vi "WrapVI.vi"() -> ()   [LabVIEW 2021]
uses:
  <vilib>/Utility/miscctls.llb/LVPositionTypeDef.ctl
panel:
  out "Facade Library Path":path=path "C:/Repositories/LVOS/jsontext Facade/lv-src/jsontext.facade.lvlib"
  in  "source VI":path
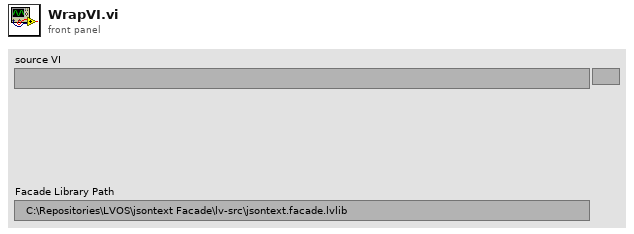
[diagram p1: front panel]
types:
  T1 = typedef "LVPositionTypeDef.ctl" = cluster{"Left":i32, "Top":i32}
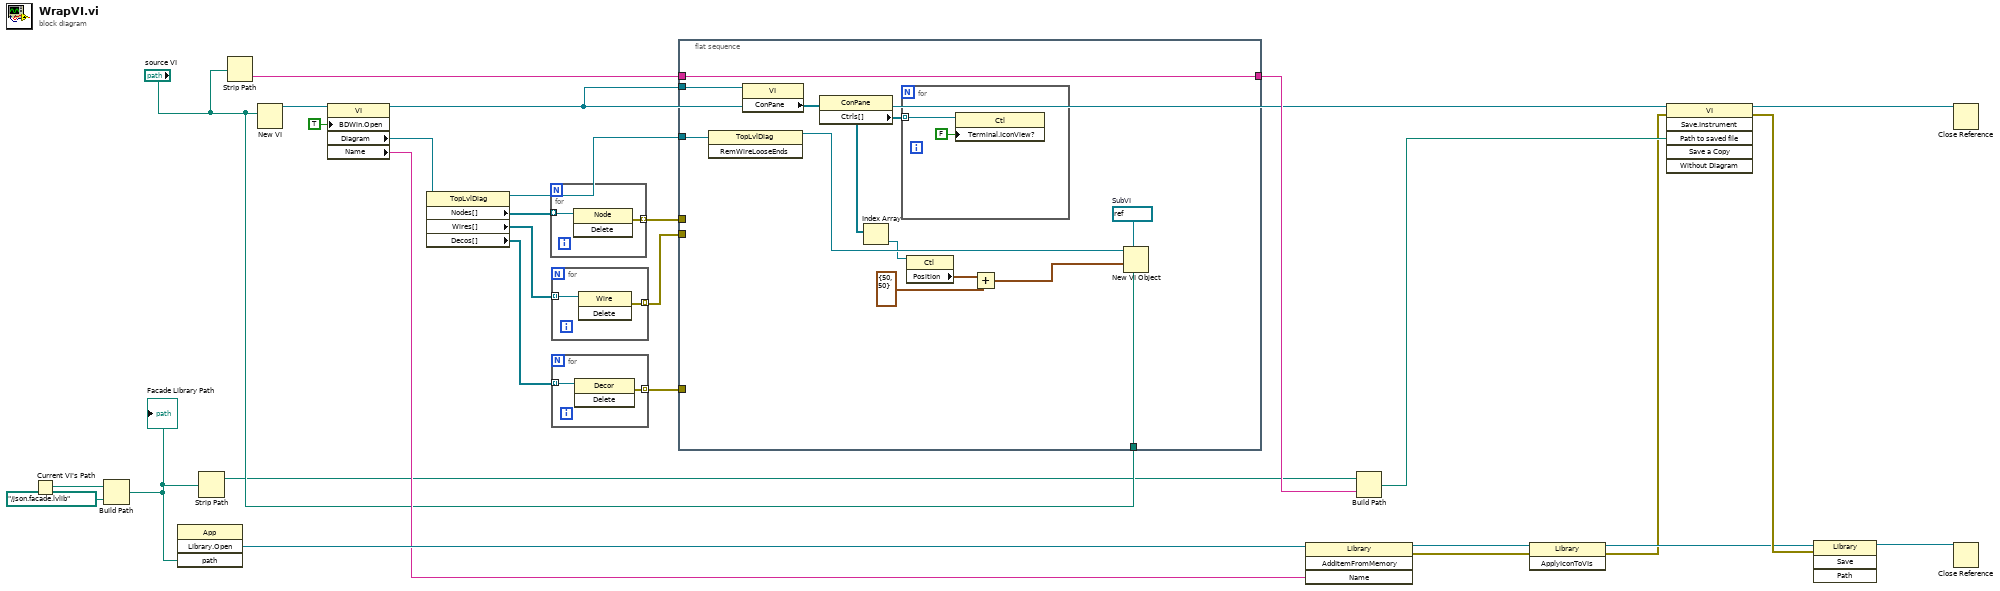
[diagram p0: block diagram]
diagram:
  n1 = Current VI's Path() -> (path=w3:path)
  n2 = Build Path(base path=w3, name or relative path=path "../json.facade.lvlib") -> (appended path=w1:path)
  "Facade Library Path" <- w1
  n3 = invoke class="App" method="Library.Open"("path"=w1) -> ("Open Library"=w26:refnum<vi>)  [unwired: 3 in, 3 out]
  n4 = Strip Path(path=w1) -> (stripped path=w4:path)  [unwired: 1 out]
  n5 = Strip Path(path="source VI") -> (name=w10:string)  [unwired: 1 out]
  n6 = New VI(10:"source VI") -> (3:w28:refnum<vi>)  [unwired: 6 in, 1 out]
  n7 = property class="VI"(reference=w28, "BDWin.Open"=TRUE ("Block Diagram Window:Open")) -> (reference out=w7:refnum<vi>, "Diagram"=w17:refnum<vi>, "Name"=w9:string)  [unwired: 1 in, 1 out]
  n8 = property class="TopLvlDiag"(reference=w17) -> (reference out=w14:refnum<vi>, "Nodes[]"=w16:refnum<vi>[], "Wires[]"=w15:refnum<vi>[], "Decos[]"=w6:refnum<vi>[])  [unwired: 1 in, 1 out]
  n9 = for {
    tunnel: w16 -> [w30] mode=indexing
    tunnel: [w29] -> w13 mode=indexing
    n10 = invoke class="Node" method="Delete"(reference=w30) -> (error out=w29:errorcluster)  [unwired: 2 in, 2 out]
  }
  n11 = for {
    tunnel: w15 -> [w32] mode=indexing
    tunnel: [w31] -> w12 mode=indexing
    n12 = invoke class="Wire" method="Delete"(reference=w32) -> (error out=w31:errorcluster)  [unwired: 2 in, 2 out]
  }
  n13 = for {
    tunnel: w6 -> [w34] mode=indexing
    tunnel: [w33] -> w5 mode=indexing
    n14 = invoke class="Decor" method="Delete"(reference=w34) -> (error out=w33:errorcluster)  [unwired: 2 in, 2 out]
  }
  n15 = flat-sequence {
    tunnel: w14 -> [w36]
    tunnel: w13 -> [_]
    tunnel: w12 -> [_]
    tunnel: [w46] -> w11
    tunnel: w10 -> [w46]
    tunnel: "source VI" -> [w44]
    tunnel: w7 -> [w43]
    tunnel: w5 -> [_]
    frame #0 {
      w45 = refnum<vi> refnum  # SubVI
      n16 = invoke class="TopLvlDiag" method="RemWireLooseEnds"(reference=w36) -> (reference out=w40:refnum<vi>)  [unwired: 2 in, 2 out]
      n17 = property class="VI"(reference=w43) -> ("ConPane"=w42:refnum<vi>)  [unwired: 1 in, 2 out]
      n18 = property class="ConPane"(reference=w42) -> ("Ctrls[]"=w41:refnum<vi>[])  [unwired: 1 in, 2 out]
      n19 = Index Array(array=w41) -> (element=w39:refnum<vi>)  [unwired: 1 in]
      n20 = for {
        tunnel: w41 -> [w48] mode=indexing
        n21 = property class="Ctl"(reference=w48, "Terminal.IconView?"=FALSE ("Terminal.Icon View?")) -> ()  [unwired: 1 in, 2 out]
      }
      n22 = property class="Ctl"(reference=w39) -> ("Position"=w38:T1)  [unwired: 1 in, 2 out]
      n23 = Add(x=w38, y=T1 {"Left"=50, "Top"=50}) -> (x+y=w35:T1)
      n24 = New VI Object(vi object class=w45, owner refnum=w40, position/next to=w35, 6:w44) -> ()  [unwired: 4 in, 2 out]
    }
  }
  n25 = invoke class="Library" method="AddItemFromMemory"(reference=w26, "Name"=w9) -> (reference out=w21:refnum<vi>, error out=w19:errorcluster)  [unwired: 2 in, 2 out]
  n26 = Build Path(base path=w4, name or relative path=w11) -> (appended path=w23:path)
  n27 = invoke class="Library" method="ApplyIconToVIs"(reference=w21, error in=w19) -> (reference out=w20:refnum<vi>, error out=w18:errorcluster)  [unwired: 1 in, 1 out]
  n28 = invoke class="VI" method="Save.Instrument"(reference=w7, error in=w18, "Path to saved file"=w23) -> (reference out=w24:refnum<vi>, error out=w22:errorcluster)  [unwired: 3 in, 4 out]
  n29 = invoke class="Library" method="Save"(reference=w20, error in=w22) -> (reference out=w25:refnum<vi>)  [unwired: 2 in, 3 out]
  n30 = Close Reference(reference=w24) -> ()  [unwired: 1 in, 1 out]
  n31 = Close Reference(reference=w25) -> ()  [unwired: 1 in, 1 out]
